vi "Read RM DMA.vi"(4 "Iteration":i32, 6 "Read Values":dbl[](array[numeric]), 8 "error in":errorcluster, 9 "VMIC reference in":T2, 10 "Block descriptors":T1[](array[typedef]), 11 "Old Values":dbl[](array[numeric])) -> (0 "error out":errorcluster, 1 "VMIC reference out":T2, 2 "Read Duration":u32, 3 "Updated Values":dbl[](array[numeric]))   [LabVIEW 2019, in "RefMem DMA Engine.lvlib"]
uses:
  RefMem DMA Engine.lvlib
  Shared/Block descriptor.ctl
  Shared/RefMem DMA Shared.lvlib
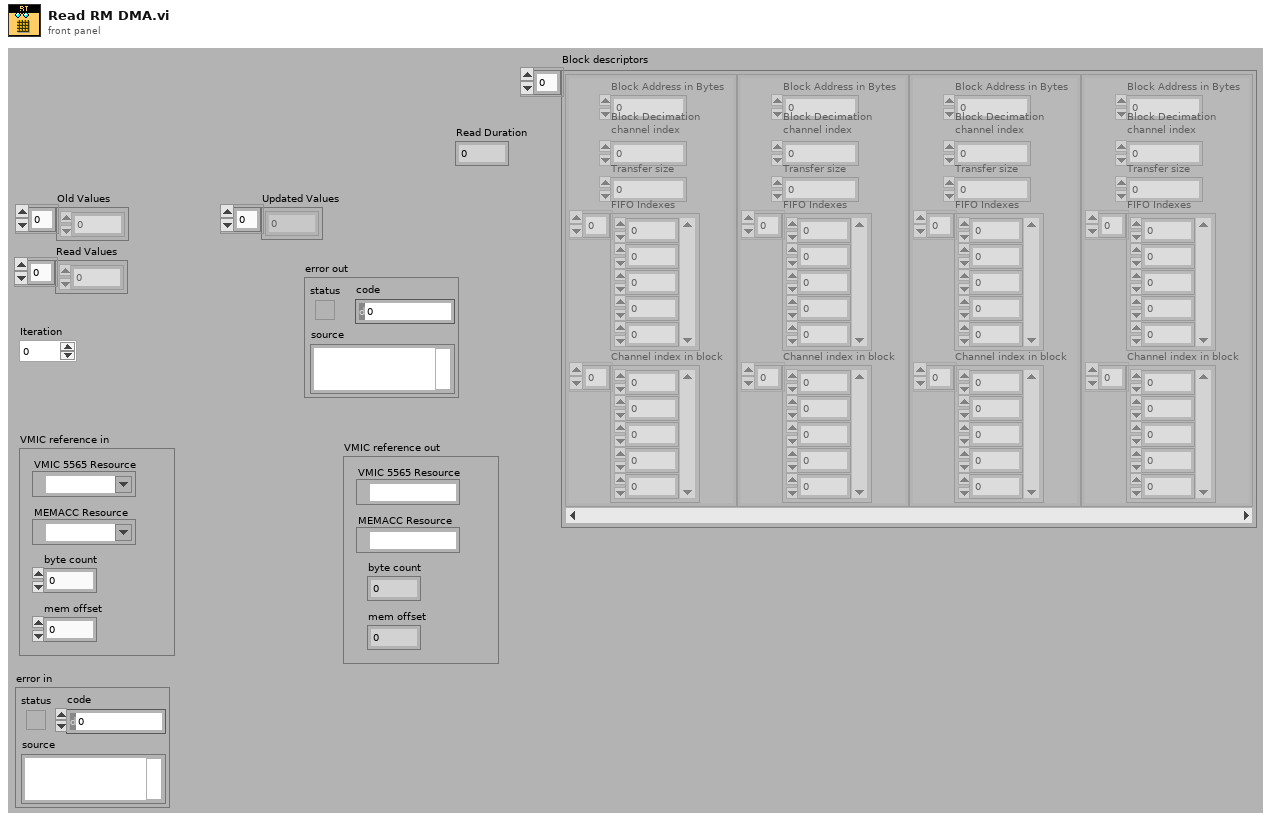
[diagram p1: front panel]
types:
  T1 = typedef "RefMem DMA Shared.lvlib/Block descriptor.ctl" = cluster{"Block Address in Bytes":u32, "Block Decimation \nchannel index":i32, "Transfer size":u32, "FIFO Indexes":i32[], "Channel index in block":i32[]}
  T2 = cluster{"VMIC 5565 Resource":refnum<visa-resource-name>, "MEMACC Resource":refnum<visa-resource-name>, "byte count":u32, "mem offset":u32}
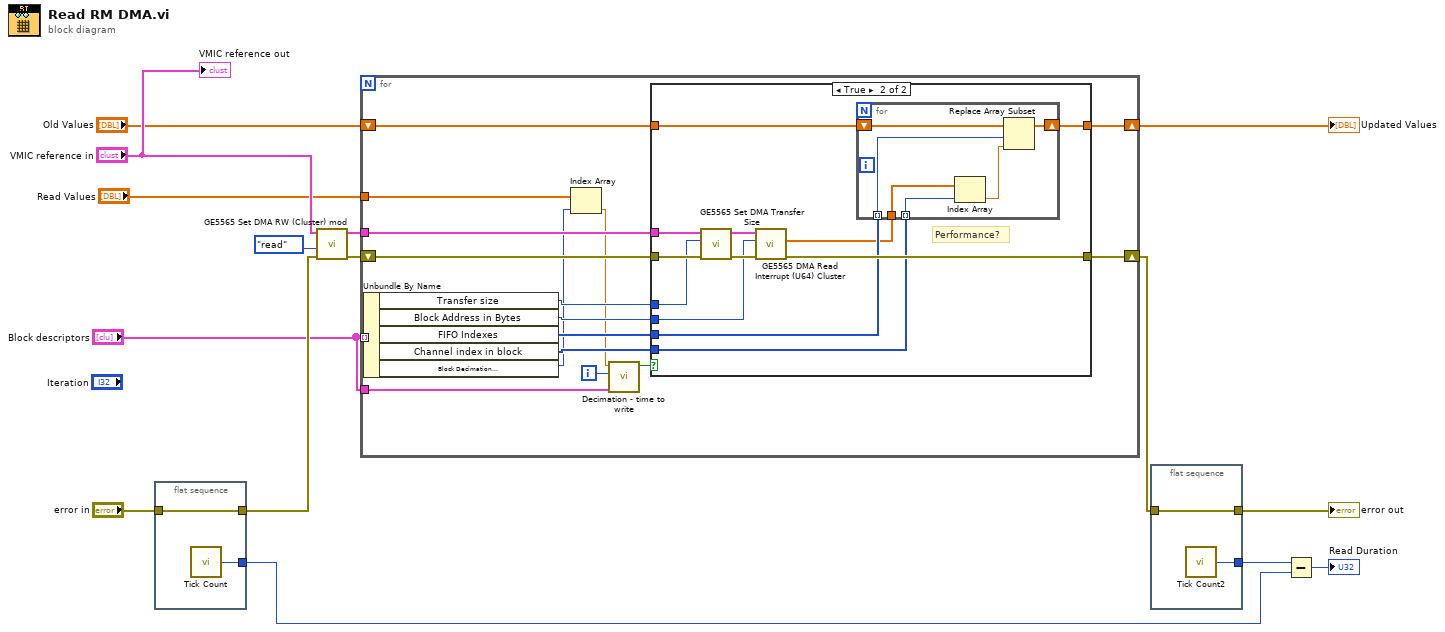
[diagram p0: block diagram]
diagram:
  n1 = flat-sequence {
    tunnel: [w17] -> w7
    tunnel: "error in" -> [w17]
    tunnel: [w16] -> w12
    frame #0 {
      n2 = call "Tick Count"() -> ("Tick Count(uSec)"=w16:u32)
    }
  }
  n3 = call "GE5565 Set DMA RW (Cluster) mod.vi"("error in (no error)"=w7, "operation (read)"=enum16{"read", "write"}."read", "VMIC-5565"="VMIC reference in") -> ("error out"=w6:errorcluster, "VMIC-5565"=w5:T2)  [unwired: 3 in]
  n4 = for "Write Output Values to System" {
    shift-right: [w30] -> w10
    shift-left: w6 -> [w32]
    shift-right: [w26] -> w3
    shift-left: "Old Values" -> [w23]
    tunnel: w5 -> [w31]
    tunnel: "Block descriptors" -> [w29] mode=indexing
    tunnel: "Read Values" -> [w20]
    tunnel: "Block descriptors" -> [w19]
    i -> [w18]
    n5 = Unbundle By Name(w29) -> ("Transfer size"=w27:u32, "Block Address in Bytes"=w28:u32, "FIFO Indexes"=w25:i32[], "Channel index in block"=w24:i32[], "Block Decimation \nchannel index"=w22:i32)
    n6 = Index Array(array=w20, index=w22) -> (element=w21:dbl)
    n7 = call "Decimation - time to write.vi"("Block descriptors"=w19, "Iteration"=w18, "Decimation"=w21) -> ("Trigger?"=w33:bool)  [unwired: 8 in]
    n8 = case shown="True" w33 {
      tunnel: [w35 w41] -> w30
      tunnel: w32 -> [w35 w47]
      tunnel: w27 -> [_ w44]
      tunnel: w28 -> [_ w43]
      tunnel: w31 -> [_ w42]
      tunnel: w23 -> [w34 w40]
      tunnel: [w34 w39] -> w26
      tunnel: w25 -> [_ w38]
      tunnel: w24 -> [_ w36]
      frame False {
      }
      frame True {
        # "Performance?"
        n9 = call "GE5565 Set DMA Transfer Size.vi"("error in (no error)"=w47, "Transfer Size"=w44, "VMIC-5565"=w42) -> ("error out"=w46:errorcluster, "VMIC-5565"=w45:T2)  [unwired: 3 in]
        n10 = call "GE5565 DMA Read Interrupt (U64) Cluster.vi"("error in (no error)"=w46, "RM offset (0)"=w43, "VMIC reference in"=w45) -> ("error out"=w41:errorcluster, "buffer"=w37:dbl[])  [unwired: 6 in, 1 out]
        n11 = for {
          tunnel: w38 -> [w51] mode=indexing
          shift-right: [w52] -> w39
          shift-left: w40 -> [w53]
          tunnel: w37 -> [w50]
          tunnel: w36 -> [w48] mode=indexing
          n12 = Index Array(array=w50, index=w48) -> (element=w49:dbl)
          n13 = Replace Array Subset(array=w53, new element=w49, index=w51) -> (w52:dbl[])
        }
      }
    }
  }
  "Updated Values" <- w3
  n14 = flat-sequence {
    tunnel: [w55] -> w14
    tunnel: w10 -> [w55]
    tunnel: [w54] -> w13
    frame #0 {
      n15 = call "Tick Count2"() -> ("Tick Count(uSec)"=w54:u32)
    }
  }
  n16 = Subtract(x=w13, y=w12) -> (x-y=→"Read Duration":u32)
  "error out" <- w14
  "VMIC reference out" <- "VMIC reference in"
